vi "sub_vi_convert_measures.vi"(0 "Mean":dbl, 2 "Standard deviation":dbl, 3 "Variance":dbl, 4 "Slope":dbl, 8 "Intercept":dbl) -> (6 "Converted mean":dbl, 7 "Converted std deviation":dbl, 9 "Converted variance":dbl)   [LabVIEW 2016]
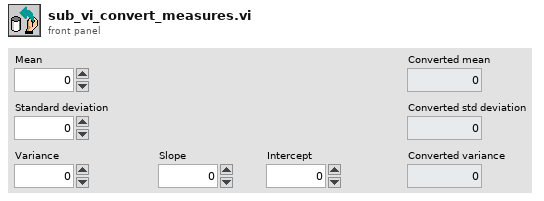
[diagram p1: front panel]
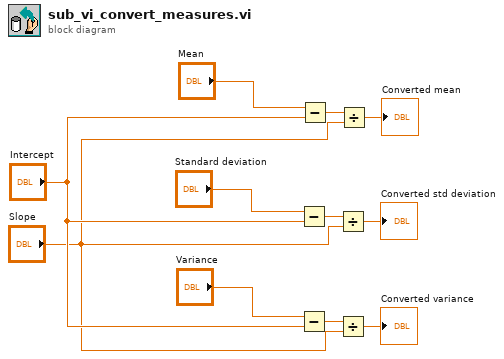
[diagram p0: block diagram]
diagram:
  n1 = Subtract(x="Standard deviation", y="Intercept") -> (x-y=w9:dbl)
  n2 = Subtract(x="Variance", y="Intercept") -> (x-y=w7:dbl)
  n3 = Subtract(x="Mean", y="Intercept") -> (x-y=w11:dbl)
  n4 = Divide(x=w9, y="Slope") -> (x/y=→"Converted std deviation":dbl)
  n5 = Divide(x=w7, y="Slope") -> (x/y=→"Converted variance":dbl)
  n6 = Divide(x=w11, y="Slope") -> (x/y=→"Converted mean":dbl)
